vi "PID vision.vi"(11 "RobotDriveDevRef in":T1={"DevStatus"={"status"=FALSE, "code"=0, "source"=""}, "Motors[]"=[], "Square Inputs"=FALSE, "Max Output"=1.0}) -> (3 "RobotDriveDevRef out":T1={"DevStatus"={"status"=FALSE, "code"=0, "source"=""}, "Motors[]"=[], "Square Inputs"=FALSE, "Max Output"=1.0})   [LabVIEW 2017]
uses:
  <vilib>/Rock Robotics/WPI/RobotDrive/WPI_RobotDriveDevRef.ctl
  <vilib>/Rock Robotics/WPI/MotorControl/WPI_MotorControlDeviceRef.ctl
  <vilib>/Rock Robotics/WPI/MotorControl/WPI_MotorControlType.ctl
  <vilib>/Rock Robotics/SystemInterfaces/DIO/FPGA_DIOPWMChannel.ctl
  <vilib>/Rock Robotics/WPI/PWM/WPI_PWMDeadband.ctl
  <vilib>/Rock Robotics/SystemInterfaces/DIO/FPGA_DIOChannel.ctl
  Robot Global Data.vi
  <vilib>/addons/control/pid/pid.llb/PID (DBL).vi
  <vilib>/addons/control/pid/NI_PID_pid.lvlib
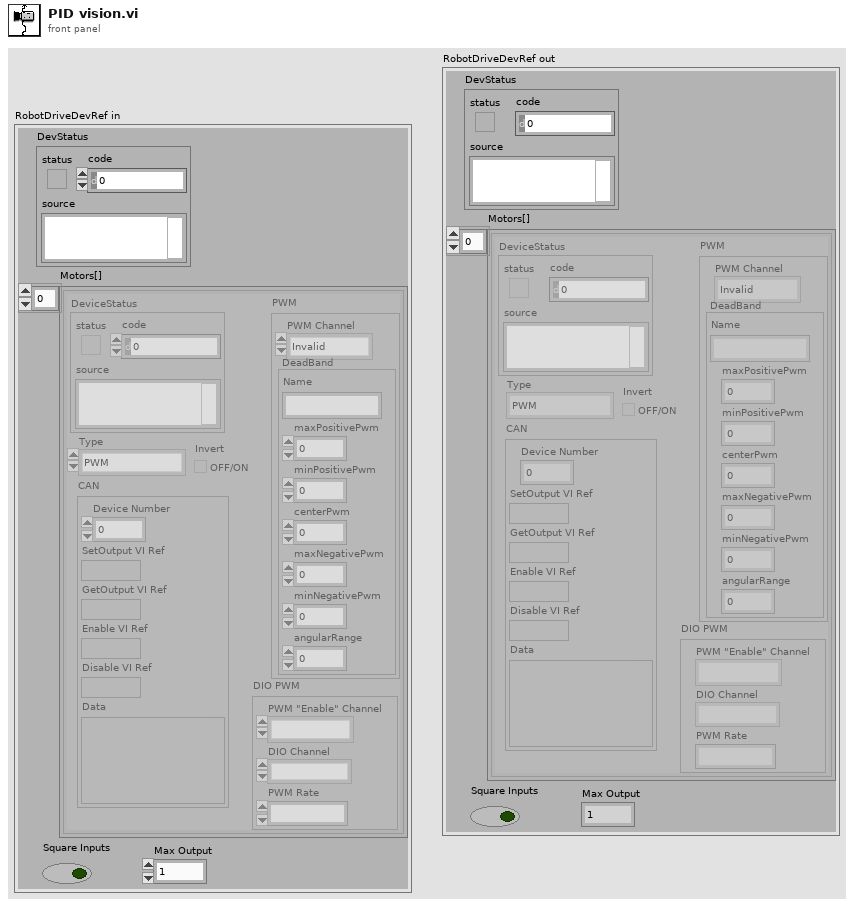
[diagram p1: front panel]
types:
  T1 = typedef "WPI_RobotDriveDevRef.ctl" = cluster{"DevStatus":errorcluster, "Motors[]":T2[], "Square Inputs":bool, "Max Output":dbl}
  T2 = typedef "WPI_MotorControlDeviceRef.ctl" = cluster{"DeviceStatus":errorcluster, "Type":T3, "PWM":cluster{"PWM Channel":T4, "DeadBand":T5}, "CAN":cluster{"Device Number":u8, "SetOutput VI Ref":variant, "GetOutput VI Ref":variant, "Enable VI Ref":variant, "Disable VI Ref":variant, "Data":variant}, "Invert":bool, "DIO PWM":cluster{"PWM \"Enable\" Channel":T4, "DIOChannel":T6, "PWM Rate":dbl}}
  T3 = typedef "WPI_MotorControlType.ctl" = enum16{"PWM", "CAN", "DIO PWM"}
  T4 = typedef "FPGA_DIOPWMChannel.ctl" = enum8{"PWM 0", "PWM 1", "PWM 2", "PWM 3", "PWM 4", "PWM 5", "PWM 6", "PWM 7", "PWM 8", "PWM 9", "PWM MXP 0", "PWM MXP 1", "PWM MXP 2", "PWM MXP 3", "PWM MXP 4", "PWM MXP 5", "PWM MXP 6", "PWM MXP 7", "PWM MXP 8", "PWM MXP 9", "Invalid"}
  T5 = typedef "WPI_PWMDeadband.ctl" = cluster{"Name":string, "maxPositivePwm":i32, "minPositivePwm":i32, "centerPwm":i32, "maxNegativePwm":i32, "minNegativePwm":i32, "angularRange":u16}
  T6 = typedef "FPGA_DIOChannel.ctl" = enum8{"DIO 0", "DIO 1", "DIO 2", "DIO 3", "DIO 4", "DIO 5", "DIO 6", "DIO 7", "DIO 8", "DIO 9", "DIO MXP 0", "DIO MXP 1", "DIO MXP 2", "DIO MXP 3", "DIO MXP 4", "DIO MXP 5", "DIO MXP 6", "DIO MXP 7", "DIO MXP 8", "DIO MXP 9", "DIO MXP 10", "DIO MXP 11", "DIO MXP 12", "DIO MXP 13", "DIO MXP 14", "DIO MXP 15", "SPI Port CS1", "SPI Port CS2", "SPI Port CS3", "SPI Port MISO", "SPI Port MOSI", "Invalid"}
  T7 = cluster{"X Center":i32, "X Tolerance":i32, "Y Center":i32, "Y Tolderance":i32}
  T8 = cluster{"CHECKSUM":u16, "SIGNATURE NUMBER":u16, "X CENTER":u16, "Y CENTER":u16, "TRAGET WIDTH":u16, "TARGET HEIGHT":u16, "X_LOCK":bool, "Y_LOCK":bool}
  T9 = cluster{"proportional gain (Kc)":dbl, "integral time (Ti, min)":dbl, "derivative time (Td, min)":dbl}
  T10 = cluster{"Motor Values[0]":dbl, "Motor Values[1]":dbl, "Motor Values[2]":dbl, "Motor Values[3]":dbl, "Motor Values[4]":dbl, "Motor Values[5]":dbl, "Motor Values[6]":dbl, "Motor Values[7]":dbl, "Motor Values[8]":dbl}
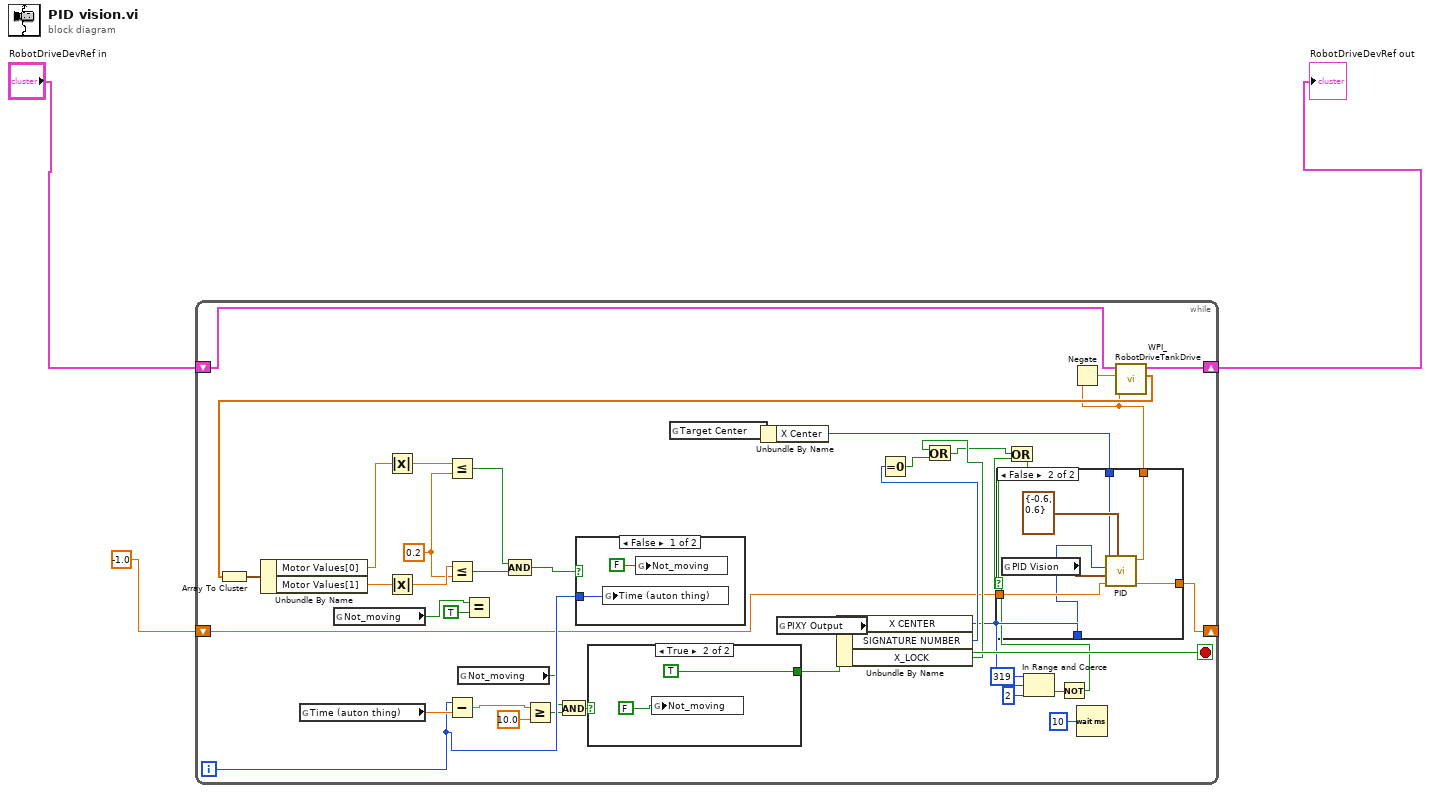
[diagram p0: block diagram]
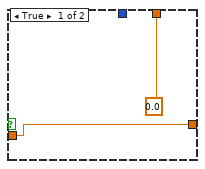
[diagram p2: hidden frame]
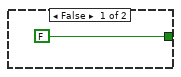
[diagram p3: hidden frame]
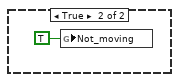
[diagram p4: hidden frame]
diagram:
  n1 = while {
    shift-right: [w42] -> w2
    shift-left: "RobotDriveDevRef in" -> [w43]
    shift-right: [w4] -> _
    shift-left: -1.0 ("dt (s)") -> [w5]
    i -> [w40]
    stop <- w34 stop-if-true
    w27 = 0.2 ("y")
    n2 = global read "Robot Global Data.vi" "Time (auton thing)"() -> (w41:dbl)
    n3 = global read "Robot Global Data.vi" "Not_moving"() -> (w26:bool)
    n4 = Subtract(x=w40, y=w41) -> (x-y=w39:dbl)
    n5 = global read "Robot Global Data.vi" "Not_moving"() -> (w36:bool)
    n6 = Equal?(x=w26, y=TRUE) -> ()  [unwired: 1 out]
    n7 = Greater Or Equal?(x=w39, y=10.0) -> (x >= y?=w37:bool)
    n8 = And(x=w36, y=w37) -> (x .and. y?=w35:bool)
    n9 = case shown="True" w35 {
      tunnel: [FALSE TRUE] -> w34
      frame False {
      }
      frame True {
        n10 = global write "Robot Global Data.vi" "Not_moving"(FALSE ("Not_moving")) -> ()
      }
    }
    n11 = global read "Robot Global Data.vi" "Target Center"() -> (w16:T7)
    n12 = Unbundle By Name(w16) -> ("X Center"=w15:i32)
    n13 = global read "Robot Global Data.vi" "PIXY Output"() -> (w20:T8)
    n14 = Unbundle By Name(w20) -> ("X CENTER"=w12:u16, "SIGNATURE NUMBER"=w17:u16, "X_LOCK"=w13:bool)
    n15 = Equal To 0?(x=w17) -> (x = 0?=w14:bool)
    n16 = Or(x=w13, y=w14) -> (x .or. y?=w9:bool)
    n17 = In Range and Coerce(upper limit=u16 319, x=w12, lower limit=u16 2) -> (In Range?=w8:bool)  [unwired: 1 out]
    n18 = Not(x=w8) -> (.not. x?=w7:bool)
    n19 = Or(x=w9, y=w7) -> (x .or. y?=w6:bool)
    n20 = case shown="False" w6 {
      tunnel: [0.0 ("output") w52] -> w18
      tunnel: w12 -> [_ w47]
      tunnel: w15 -> [_ w46]
      tunnel: w5 -> [w44 w49]
      tunnel: [w44 w48] -> w4
      frame True {
      }
      frame False {
        n21 = global read "Robot Global Data.vi" "PID Vision"() -> (w50:T9)
        n22 = call-poly <vilib>:"PID.vi"("output range"=cluster{"output high":dbl, "output low":dbl} {"output high"=-0.6, "output low"=0.6}, "dt (s)"=w49, "PID gains"=w50, "process variable"=w47, "setpoint"=w46) -> ("dt out (s)"=w48:dbl, "output"=w52:dbl)  [unwired: 5 in]
      }
    }
    n23 = Negate(x=w18) -> (-x=w19:dbl)
    n24 = Wait (ms)(milliseconds to wait=u32 10) -> ()  [unwired: 1 out]
    n25 = call <vilib>:"WPI_RobotDriveTankDrive.vi"("Right axis value"=w18, "Left axis value"=w19, "RobotDriveDevRef"=w43) -> ("Motor Values"=w33:dbl[], "RobotDriveDevRef"=w42:T1)  [unwired: 6 in, 1 out]
    n26 = Array To Cluster(array=w33) -> (cluster=w32:T10)
    n27 = Unbundle By Name(w32) -> ("Motor Values[0]"=w31:dbl, "Motor Values[1]"=w30:dbl)
    n28 = Absolute Value(x=w31) -> (abs(x)=w29:dbl)
    n29 = Absolute Value(x=w30) -> (abs(x)=w28:dbl)
    n30 = Less Or Equal?(x=w29, y=w27) -> (x <= y?=w24:bool)
    n31 = Less Or Equal?(x=w28, y=w27) -> (x <= y?=w23:bool)
    n32 = Compound Arithmetic op=AND(w24, w23) -> (w22:bool)
    n33 = case shown="False" w22 {
      tunnel: w40 -> [w56 _]
      frame False {
        n34 = global write "Robot Global Data.vi" "Time (auton thing)"(w56) -> ()
        n35 = global write "Robot Global Data.vi" "Not_moving"(FALSE ("Not_moving")) -> ()
      }
      frame True {
        n36 = global write "Robot Global Data.vi" "Not_moving"(TRUE ("Not_moving")) -> ()
      }
    }
  }
  "RobotDriveDevRef out" <- w2
